vi "Main.vi"() -> ()   [LabVIEW 2017, in "StatePatternDemo.lvclass"]
uses:
  StatePatternDemo.lvclass
  Player Class/Player.lvclass
  ConsoleOut/Print Options.ctl
  Player Class/Player.lvclass/Player.ctl
  State Class/State.lvclass
panel:
  in  "Previous Button":bool
  in  "Next Button":bool
  in  "Play Button":bool
  in  "Stop":bool
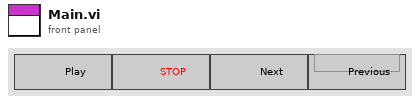
[diagram p1: front panel]
types:
  T1 = typedef "Print Options.ctl" = enum16{"Create", "Get Reference", "Print", "Print Header", "Close"}
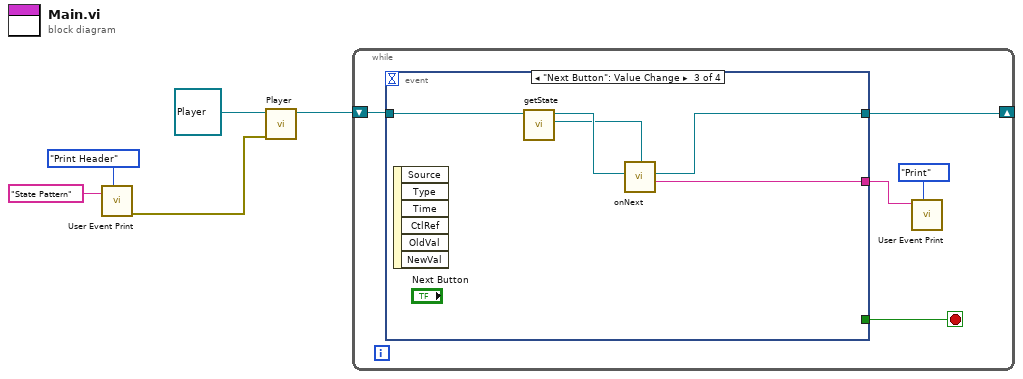
[diagram p0: block diagram]
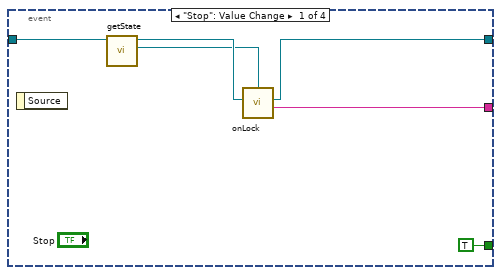
[diagram p2: hidden frame]
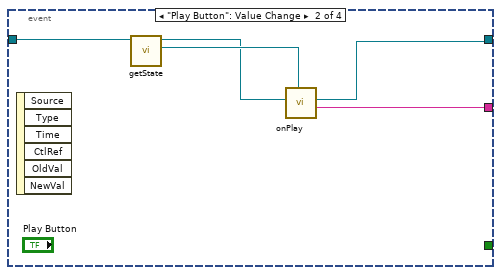
[diagram p3: hidden frame]
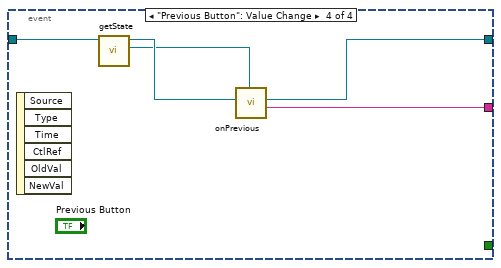
[diagram p4: hidden frame]
diagram:
  n1 = call "User Event Print.vi"("Options"=Print_Options."Print Header", "String to Print"="State Pattern") -> ("error out"=w2:errorcluster)  [unwired: 8 in, 1 out]
  n2 = call "Player.vi"("error in (no error)"=w2, "Player in"=refnum<class "Player.lvclass"> refnum ("Player.lvclass")) -> ("Player out"=w4:refnum<class "Player.lvclass">)  [unwired: 8 in, 1 out]
  n3 = while {
    shift-right: [w8] -> _
    shift-left: w4 -> [w9]
    stop <- w10 stop-if-true
    n4 = event shown="[2] \"Next Button\": Value Change" {
      selector: _ -> [_ _ _ _]
      dyn-events: _ -> [_ _ _ _]
      timeout: _ -> [_ _ _ _]
      tunnel: [TRUE _ _ _] -> w10
      tunnel: w9 -> [w15 w21 w26 w31]
      tunnel: [w13 w18 w23 w29] -> w8
      tunnel: [w11 w17 w22 w27] -> w7
      event "Stop": Value Change {
        n5 = event-data() -> ()  [unwired: 1 in, 1 out]
        n6 = call "getState.vi"("Player in"=w15) -> ("State.lvclass"=w12:refnum<class "State.lvclass">, "Player out"=w14:refnum<class "Player.lvclass">)  [unwired: 8 in, 1 out]
        n7 = call-dynamic "onLock.vi"("Player In"=w14, "State in"=w12) -> ("String"=w11:string, "Player Out"=w13:refnum<class "Player.lvclass">)  [unwired: 6 in, 2 out]
      }
      event "Play Button": Value Change {
        n8 = event-data() -> ()  [unwired: 1 in, 6 out]
        n9 = call "getState.vi"("Player in"=w21) -> ("State.lvclass"=w20:refnum<class "State.lvclass">, "Player out"=w19:refnum<class "Player.lvclass">)  [unwired: 8 in, 1 out]
        n10 = call-dynamic "onPlay.vi"("Player In"=w19, "State in"=w20) -> ("String"=w17:string, "Player Out"=w18:refnum<class "Player.lvclass">)  [unwired: 6 in, 2 out]
      }
      event "Next Button": Value Change {
        n11 = event-data() -> ()  [unwired: 1 in, 6 out]
        n12 = call "getState.vi"("Player in"=w26) -> ("State.lvclass"=w24:refnum<class "State.lvclass">, "Player out"=w25:refnum<class "Player.lvclass">)  [unwired: 8 in, 1 out]
        n13 = call-dynamic "onNext.vi"("Player In"=w25, "State in"=w24) -> ("String"=w22:string, "Player Out"=w23:refnum<class "Player.lvclass">)  [unwired: 6 in, 2 out]
      }
      event "Previous Button": Value Change {
        n14 = event-data() -> ()  [unwired: 1 in, 6 out]
        n15 = call "getState.vi"("Player in"=w31) -> ("State.lvclass"=w28:refnum<class "State.lvclass">, "Player out"=w30:refnum<class "Player.lvclass">)  [unwired: 8 in, 1 out]
        n16 = call-dynamic "onPrevious.vi"("Player In"=w30, "State in"=w28) -> ("String"=w27:string, "Player Out"=w29:refnum<class "Player.lvclass">)  [unwired: 6 in, 2 out]
      }
    }
    n17 = call "User Event Print.vi"("Options"=Print_Options."Print", "String to Print"=w7) -> ()  [unwired: 8 in, 2 out]
  }
